vi "Lissajous with Express VIs.vi"() -> ()   [LabVIEW 2023]
doc: "This example shows a Lissajous curve in an X/Y Graph. \n\nChoose the raw frequencies for X and Y and trim the movement with the Trim Slider.\n\nThis example uses the following Express VIs: Formula, Simulate Signal, and Build XY Graph."
uses:
  Instance           3 17Saved   Lissajous .vi
  Instance           2 17Saved   Lissajous .vi
  <vilib>/express/express arith-compare/Formula/XNode/ExpressFormulaBlockNode.xnode
panel:
  in  "Y":i32(slide)=3 scale=0.0..10.0
  in  "Trim":dbl(slide)=0.09048723897911828 scale=-1.0..1.0
  in  "X":i32(slide)=4 scale=0.0..10.0
  out "XY Graph":cluster{"Y":dbl[], "Y":dbl[]}[](graph)
  in  "Stop":bool
  # "Overview: Shows a Lissajous curve in an XY Graph.\nInstructions:\n1. Run the VI.\n2. Choose the raw frequencies for X and Y.\n3. Trim the movement with the Trim slider.\n4. Click Stop to stop the VI."
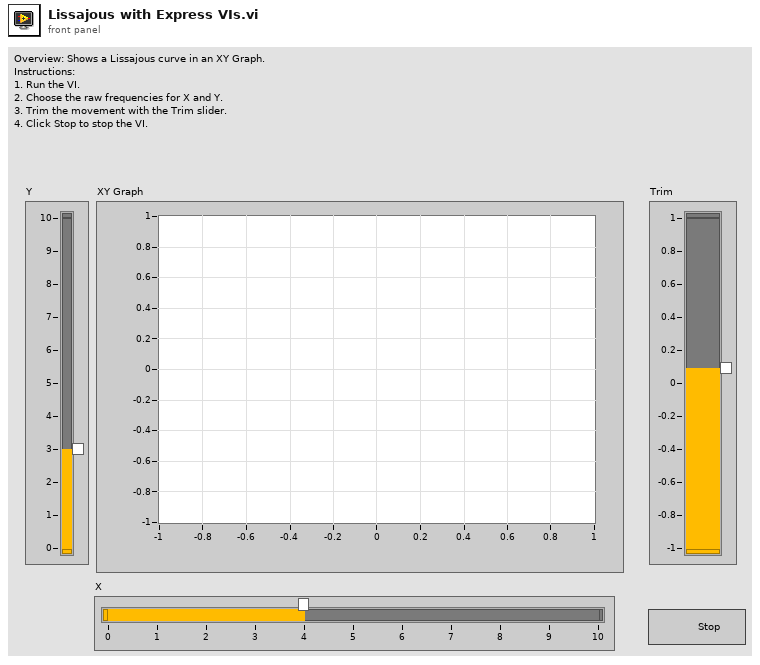
[diagram p1: front panel]
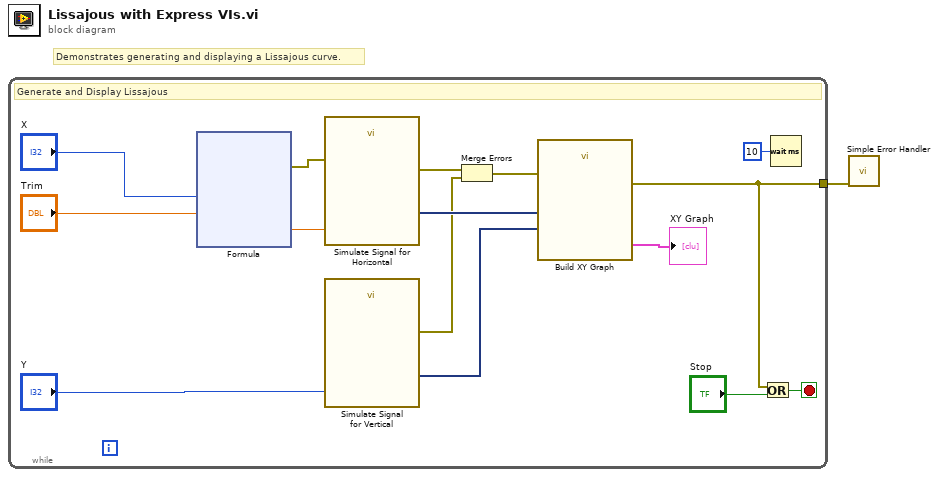
[diagram p0: block diagram]
diagram:
  # "Demonstrates generating and displaying a Lissajous curve."
  n1 = while {
    tunnel: [w2] -> w1
    stop <- w5 stop-if-true
    # "Generate and Display Lissajous"
    n2 = xnode "Formula"("X"="X", "Trim"="Trim") -> ("Result"=w13:dbl, "error out"=w7:errorcluster)  [unwired: 1 in]
    n3 = call "Simulate Signal for Horizontal"("Frequency"=w13, "error in (no error)"=w7) -> ("Sine"=w12:dynamicdata, "error out"=w6:errorcluster)  [unwired: 4 in, 8 out]
    n4 = call "Simulate Signal\nfor Vertical"("Frequency"="Y") -> ("Sine"=w11:dynamicdata, "error out"=w3:errorcluster)  [unwired: 5 in, 8 out]
    n5 = Merge Errors(w6, w3) -> (w4:errorcluster)
    n6 = call "Build XY Graph"("error in (no error)"=w4, "Y Input"=w11, "X Input"=w12) -> ("error out"=w2:errorcluster, "XY Graph"=→"XY Graph":cluster{"Y":dbl[], "Y":dbl[]}[])  [unwired: 2 in, 5 out]
    n7 = Or(x=w2, y="Stop") -> (x .or. y?=w5:bool)
    n8 = Wait (ms)(milliseconds to wait=u32 10) -> ()  [unwired: 1 out]
  }
  n9 = call <vilib>:"Simple Error Handler.vi"("error in (no error)"=w1) -> ()  [unwired: 4 in, 5 out]
